vi "Module Loop Constructor.vi"(8 "error in (no error)":errorcluster, 10 "Name":string, 11 "Type":string) -> (0 "error out":errorcluster, 3 "Module Loop.lvclass":refnum<class "Module Loop.lvclass">)   [LabVIEW 2025, in "Module Loop.lvclass"]
doc: "Instantiate instance of loop type with name."
uses:
  Module Loop.lvclass
  Digital High Speed Loop/Digital High Speed Loop.lvclass
  Structures/Structures.lvclass/Structures.ctl
  Structures/Write Name.vi
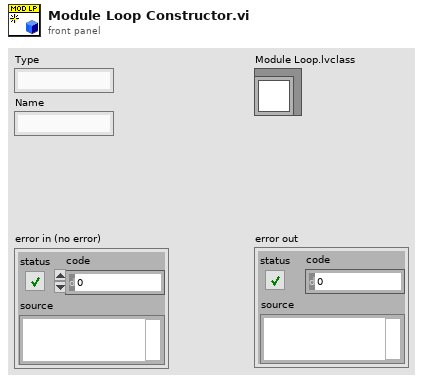
[diagram p1: front panel]
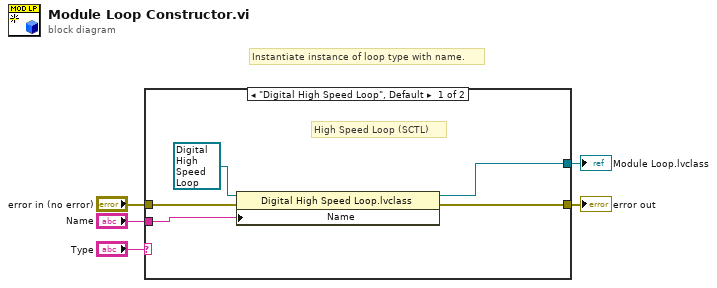
[diagram p0: block diagram]
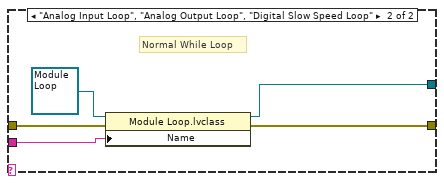
[diagram p2: hidden frame]
diagram:
  # "Instantiate instance of loop type with name."
  n1 = case shown="\"Digital High Speed Loop\", Default" "Type" {
    tunnel: [w7 w14] -> w4
    tunnel: "Name" -> [w6 w13]
    tunnel: "error in (no error)" -> [w10 w12]
    tunnel: [w8 w11] -> w1
    frame "Digital High Speed Loop", Default {
      # "High Speed Loop (SCTL)"
      n2 = property class="Digital High Speed Loop.lvclass"(reference=refnum<class "Digital High Speed Loop.lvclass"> refnum ("Digital High Speed Loop.lvclass"), error in=w10, "Name"=w6) -> (reference out=w8:refnum<class "Digital High Speed Loop.lvclass">, error out=w7:errorcluster)
    }
    frame "Analog Input Loop", "Analog Output Loop", "Digital Slow Speed Loop" {
      # "Normal While Loop"
      n3 = property class="Module Loop.lvclass"(reference=refnum<class "Module Loop.lvclass"> refnum ("Module Loop.lvclass"), error in=w12, "Name"=w13) -> (reference out=w11:refnum<class "Module Loop.lvclass">, error out=w14:errorcluster)
    }
  }
  "error out" <- w4
  "Module Loop.lvclass" <- w1
